vi "NI VeriStand - Get Custom Device Channel List.vi"(7 "Channel Type":T1, 8 "error in (no error)":errorcluster, 11 "Device Ref in":T2 format="%.0x") -> (0 "error out":errorcluster, 2 "Specified Channel Ref List":T2[](array[typedef]) format="%.0x", 3 "Device Ref out":T2 format="%.0x")   [LabVIEW 2019, in "Custom Device API.lvlib"]
doc: "Returns an array of references to all the input or output channels of a custom device."
uses:
  Custom Device API.lvlib
  Custom Device Item Ref.ctl
  Custom Device Channel Type.ctl
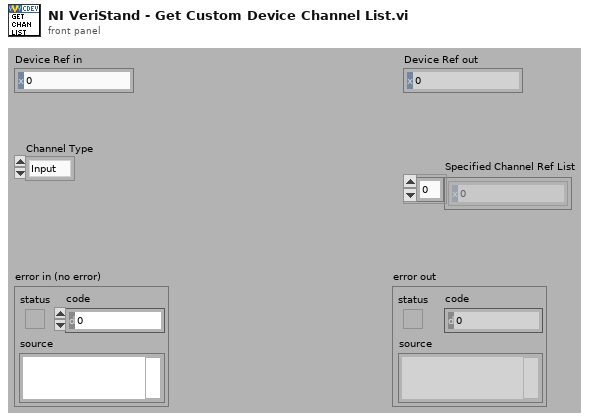
[diagram p1: front panel]
types:
  T1 = typedef "Custom Device API.lvlib/Custom Device Channel Type.ctl" = enum16{"Input", "Output"}
  T2 = typedef "Custom Device API.lvlib/Custom Device Item Ref.ctl" = u64
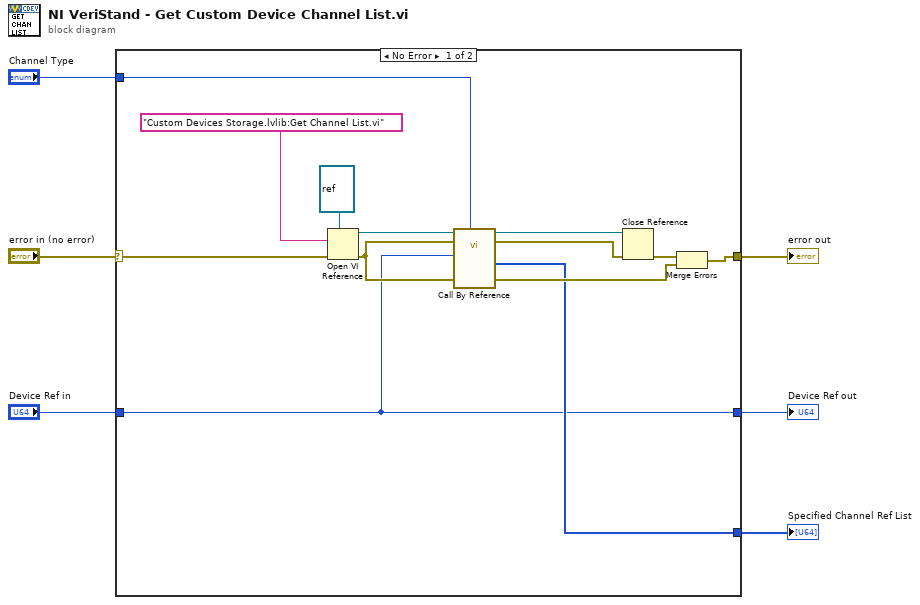
[diagram p0: block diagram]
diagram:
  n1 = case shown="No Error" "error in (no error)" {
    selector: "error in (no error)" -> [w8 w21]
    tunnel: [w11 w21] -> w6
    tunnel: "Device Ref in" -> [w7 w20]
    tunnel: "Channel Type" -> [w10 _]
    tunnel: [w7 w20] -> w3
    tunnel: [w9 _] -> w2
    frame No Error {
      n2 = Open VI Reference(type specifier VI Refnum (for type only)=refnum<vi> refnum, vi path="Custom Devices Storage.lvlib:Get Channel List.vi", error in (no error)=w8) -> (vi reference=w16:refnum<vi>, error out=w19:errorcluster)  [unwired: 3 out]
      n3 = call-by-ref "?"(reference=w16, error in=w19, "Channel Type"=w10, 8:"error in (no error)"=w19, "Device Ref in"=w7) -> (reference out=w13:refnum<vi>, error out=w14:errorcluster, 0:"error out"=w15:errorcluster, "Specified Channel Ref List"=w9:T2[])  [unwired: 6 in, 1 out]
      n4 = Close Reference(reference=w13, error in (no error)=w14) -> (error out=w12:errorcluster)
      n5 = Merge Errors(w12, w15) -> (w11:errorcluster)
    }
    frame Error {
    }
  }
  "Device Ref out" <- w3
  "error out" <- w6
  "Specified Channel Ref List" <- w2
